vi "Fetch VI Method Info.vi"(8 "Error in":errorcluster caption="Error in (no error)", 9 "Dispatch (None)":T4, 10 "VI Reference":refnum<vi>, 11 "VI ProjectItem in":refnum<vi>) -> (0 "Error out":errorcluster, 3 "Method Spec Cluster":T1)   [LabVIEW 2023, in "VIDoc Parsing.lvlib"]
uses:
  VIDoc Parsing.lvlib
  TypeDefs/Class Dispatch Type Enum.ctl
  TypeDefs/Method Spec Cluster.ctl
  TypeDefs/VI Type Extended Enum.ctl
  <vilib>/picture/picture.llb/imagedata.ctl
  TypeDefs/Controls Info Cluster.ctl
  <vilib>/Utility/miscctls.llb/LVKeyTypeDef.ctl
  <vilib>/Utility/miscctls.llb/LVPointTypeDef.ctl
  Structure Reporter/Tree Cluster.ctl
  Structure Reporter/Structure Reporter.lvlib
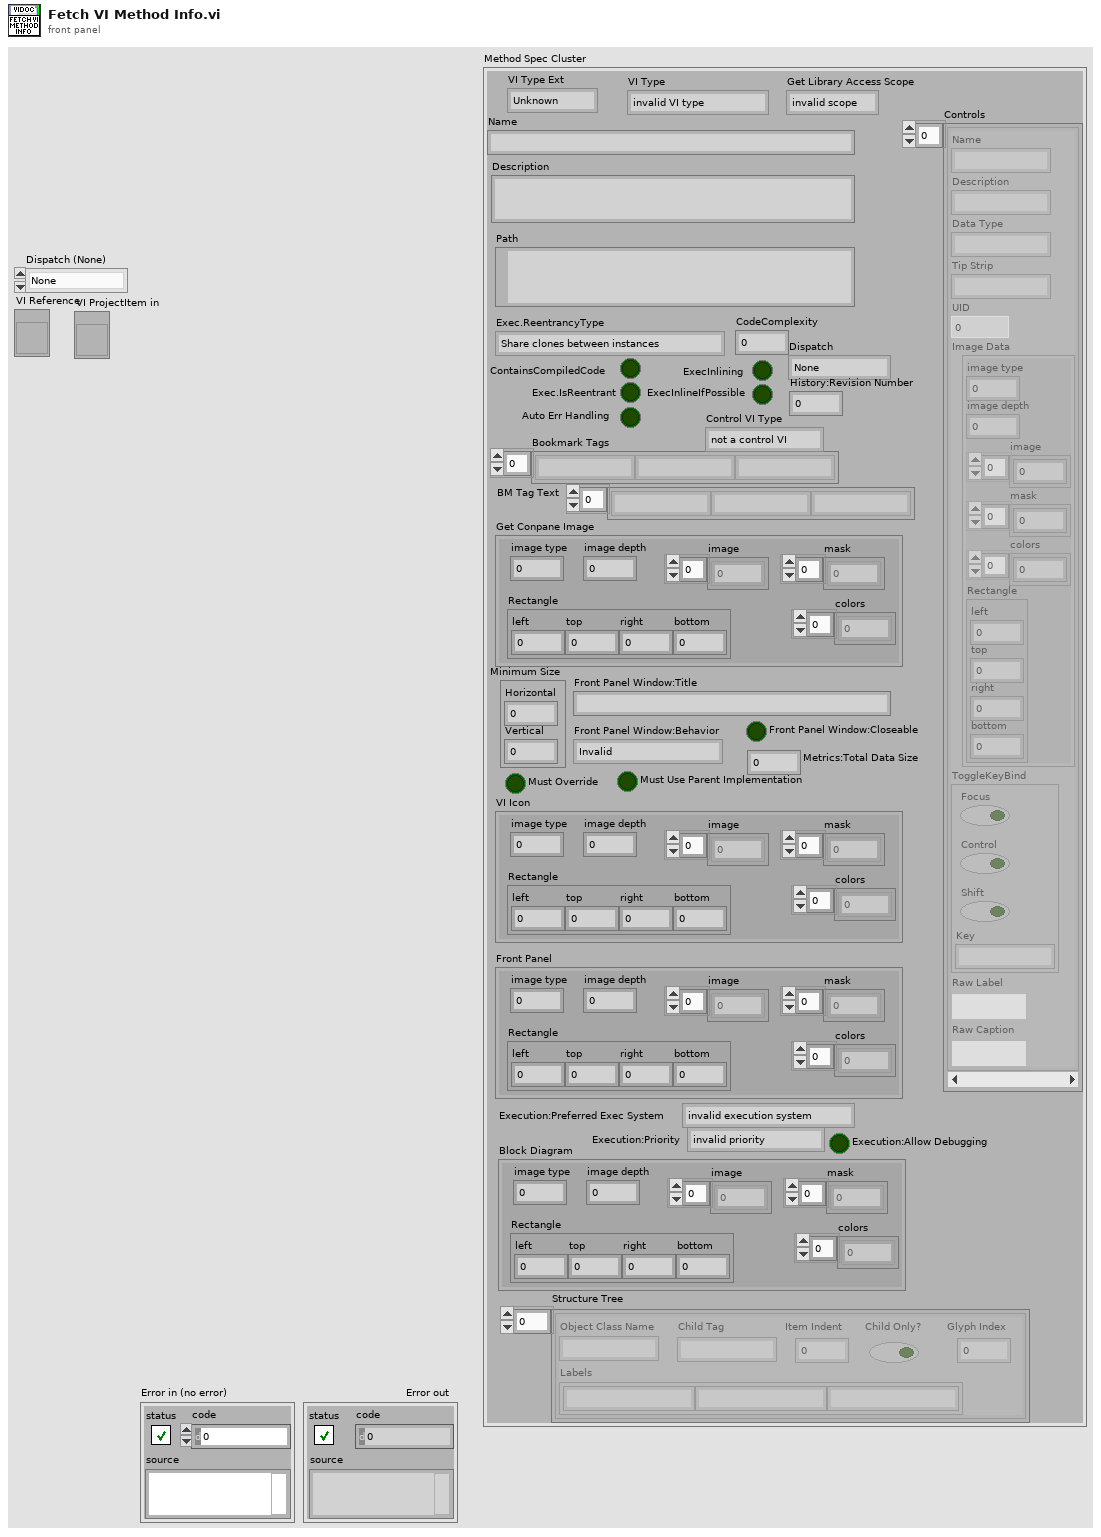
[diagram p1: front panel]
types:
  T1 = typedef "VIDoc Parsing.lvlib/Method Spec Cluster.ctl" = cluster{"VI Type Ext":T2, "Name":string, "Path":path, "Get Conpane Image":T3, "Description":string, "Get Library Access Scope":enum32{"invalid scope", "public", "private", "protected", "community"}, "Dispatch":T4, "ContainsCompiledCode":bool, "Exec.IsReentrant":bool, "Exec.ReentrancyType":enum16{"Share clones between instances", "Preallocate clone for each instance"}, "ExecInlining":bool, "ExecInlineIfPossible":bool, "Auto Err Handling":bool, "CodeComplexity":sgl, "Bookmark Tags":string[], "Control VI Type":enum32{"not a control VI", "control", "typedef", "strict typedef"}, "Controls":T5[], "VI Type":enum32{"invalid VI type", "Standard VI", "Control VI", "Global VI", "Polymorphic VI", "Configuration VI", "SubSystem", "Facade VI", "Method VI", "Statechart Diagram VI"}, "Minimum Size":T7, "Front Panel Window:Title":string, "Front Panel Window:Behavior":enum32{"Invalid", "Default", "Floating", "Floating/Auto-Hide", "Modal"}, "Front Panel Window:Closeable":bool, "Must Override":bool, "Must Use Parent Implementation":bool, "VI Icon":T3, "Front Panel":T3, "History:Revision Number":u32, "Metrics:Total Data Size":u32, "Execution:Allow Debugging":bool, "Execution:Preferred Exec System":enum32{"invalid execution system", "user interface", "standard", "instrument i/o", "data acquisition", "other 1", "other 2", "same as caller"}, "Execution:Priority":enum32{"invalid priority", "background priority", "normal priority", "above normal priority", "high priority", "time critical priority", "subroutine"}, "BM Tag Text":string[], "Block Diagram":T3, "Structure Tree":T8[]}
  T2 = typedef "VIDoc Parsing.lvlib/VI Type Extended Enum.ctl" = enum16{"Unknown", "Class Method", "Class Accessor Get", "Class Accessor Set", "Class Control", "Library Method", "Library Control", "VI", "Control"}
  T3 = typedef "imagedata.ctl" = cluster{"image type":i32, "image depth":i32, "image":u8[], "mask":u8[], "colors":u32[], "Rectangle":cluster{"left":i16, "top":i16, "right":i16, "bottom":i16}}
  T4 = typedef "VIDoc Parsing.lvlib/Class Dispatch Type Enum.ctl" = enum16{"None", "Static", "Dynamic"}
  T5 = typedef "VIDoc Parsing.lvlib/Controls Info Cluster.ctl" = cluster{"Name":string, "Description":string, "Data Type":string, "Tip Strip":string, "UID":i32, "Image Data":T3, "ToggleKeyBind":T6, "Raw Label":string, "Raw Caption":string}
  T6 = typedef "LVKeyTypeDef.ctl" = cluster{"Focus":bool, "Control":bool, "Shift":bool, "Key":string}
  T7 = typedef "LVPointTypeDef.ctl" = cluster{"Horizontal":i16, "Vertical":i16}
  T8 = typedef "VIDoc Parsing.lvlib/Structure Reporter.lvlib/Tree Cluster.ctl" = cluster{"Object Class Name":string, "Labels":string[], "Child Tag":string, "Item Indent":i32, "Child Only?":bool, "Glyph Index":i32}
  T9 = enum32{"not a control VI", "control", "typedef", "strict typedef"}
  T10 = enum16{"Share clones between instances", "Preallocate clone for each instance"}
  T11 = enum32{"invalid execution system", "user interface", "standard", "instrument i/o", "data acquisition", "other 1", "other 2", "same as caller"}
  T12 = enum32{"invalid priority", "background priority", "normal priority", "above normal priority", "high priority", "time critical priority", "subroutine"}
  T13 = enum32{"invalid scope", "public", "private", "protected", "community"}
  T14 = typedef "VIDoc Parsing.lvlib/Structure Reporter.lvlib/Structure Result 2.ctl" = cluster{"Depth":i32, "Top":i32, "Left":i32, "Frame index":i32, "Struct":i32, "Object Class Name":string, "Object UID":i32, "Label Visible":bool, "Object Label":string, "SD Label Visible":bool, "Object SD Label":string, "Frame Name":string, "Diag UID":i32, "Owner Class Name":string, "Owner UID":i32, "Diag Struct":i32[], "Parent Struct":i32, "Diag UIDs":i32[], "Tree Name":string, "Diag Ref":refnum<vi>, "Owner Classes":string[], "Owner":refnum<vi>, "Owner UIDs":i32[], "Tag Indent":i32, "Tag Value":i32, "Child Tag":string}
  T15 = typedef "LVBookmarkInfoTypeDef.ctl" = cluster{"Bookmark ID":u32, "Bookmark Tag":string, "Label Text":string}[]
  T16 = enum32{"Invalid", "Default", "Floating", "Floating/Auto-Hide", "Modal"}
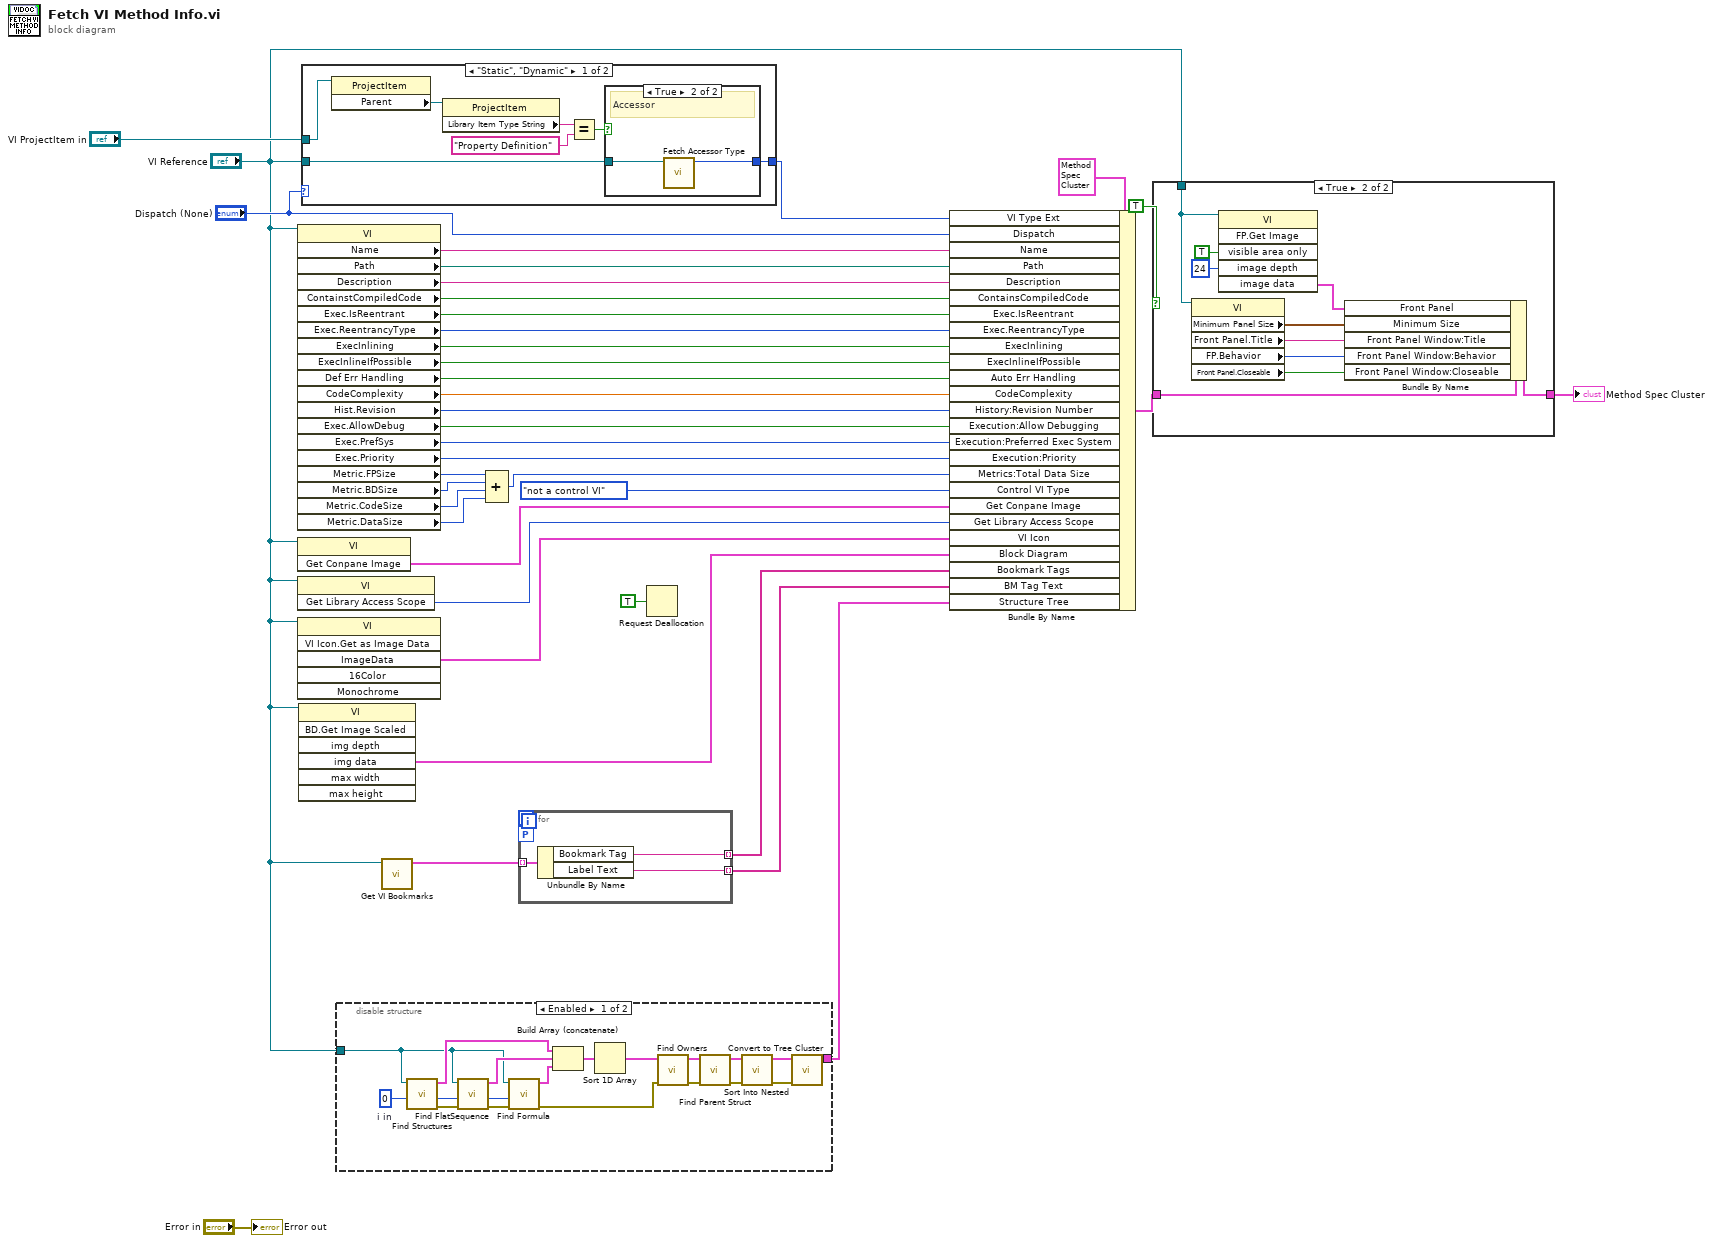
[diagram p0: block diagram]
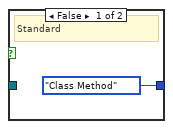
[diagram p4: hidden frame]
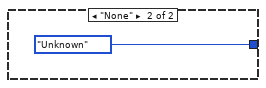
[diagram p5: hidden frame]
diagram:
  n1 = property class="VI"(reference="VI Reference") -> ("Name"=w31:string, "Path"=w30:path, "Description"=w29:string, "ContainstCompiledCode"=w28:bool, "Exec.IsReentrant"=w27:bool, "Exec.ReentrancyType"=w26:T10, "ExecInlining"=w25:bool, "ExecInlineIfPossible"=w24:bool, "Def Err Handling"=w23:bool, "CodeComplexity"=w22:sgl, "Hist.Revision"=w21:u32, "Exec.AllowDebug"=w20:bool, "Exec.PrefSys"=w19:T11, "Exec.Priority"=w18:T12, "Metric.FPSize"=w36:u32, "Metric.BDSize"=w35:u32, "Metric.CodeSize"=w34:u32, "Metric.DataSize"=w33:u32)  [unwired: 1 in, 2 out]
  n2 = invoke class="VI" method="Get Conpane Image"(reference="VI Reference") -> ("Get Conpane Image"=w16:T3)  [unwired: 2 in, 2 out]
  n3 = invoke class="VI" method="Get Library Access Scope"(reference="VI Reference") -> ("Get Library Access Scope"=w15:T13)  [unwired: 2 in, 2 out]
  n4 = invoke class="VI" method="VI Icon.Get as Image Data"(reference="VI Reference") -> ("ImageData"=w14:T3)  [unwired: 5 in, 5 out]
  n5 = invoke class="VI" method="BD.Get Image Scaled"(reference="VI Reference") -> ("img data"=w4:T3)  [unwired: 6 in, 6 out]
  n6 = case shown="\"Static\", \"Dynamic\"" "Dispatch (None)" {
    tunnel: "VI ProjectItem in" -> [w45 _]
    tunnel: [w41 VI_Type_Extended_Enum."Unknown" ("VI Type Ext")] -> w11
    tunnel: "VI Reference" -> [w39 _]
    frame "Static", "Dynamic" {
      n7 = property class="ProjectItem"(reference=w45) -> ("Parent"=w42:refnum<vi>)  [unwired: 1 in, 2 out]
      n8 = property class="ProjectItem"(reference=w42) -> ("Library Item Type String"=w43:string)  [unwired: 1 in, 2 out]
      n9 = Equal?(x=w43, y="Property Definition") -> (x = y?=w40:bool)
      n10 = case shown="True" w40 {
        tunnel: [VI_Type_Extended_Enum."Class Method" w47] -> w41
        tunnel: w39 -> [_ w48]
        frame False {
          # "Standard"
        }
        frame True {
          # "Accessor"
          n11 = call "Fetch Accessor Type.vi"("VI in"=w48) -> ("VI Type Ext"=w47:T2)  [unwired: 9 in, 1 out]
        }
      }
    }
    frame "None" {
    }
  }
  n12 = disable-structure "Diagram Disable Structure" shown="Enabled" {
    disable-tunnel: [w54 _] -> w3
    disable-tunnel: "VI Reference" -> [w50 _]
    frame Enabled {
      w67 = 0  # i in
      n13 = call "Find Structures.vi"("i in"=w67, "VI in"=w50) -> ("error out"=w53:errorcluster, "i out"=w66:i32, "Structures"=w68:T14[])  [unwired: 7 in]
      n14 = call "Find FlatSequence.vi"("error in (no error)"=w53, "i in"=w66, "VI in"=w50) -> ("error out"=w52:errorcluster, "i out"=w63:i32, "FlatSequences"=w65:T14[])  [unwired: 6 in]
      n15 = call "Find Formula.vi"("error in (no error)"=w52, "i in"=w63, "VI in"=w50) -> ("error out"=w51:errorcluster, "Array"=w64:T14[])  [unwired: 6 in, 1 out]
      n16 = Build Array (concatenate)(w68, w65, w64) -> (w62:T14[])
      n17 = Sort 1D Array(array=w62) -> (sorted array=w61:T14[])
      n18 = call "Find Owners.vi"("error in (no error)"=w51, "Array in"=w61) -> ("error out"=w59:errorcluster, "Array out"=w60:T14[])  [unwired: 8 in]
      n19 = call "Find Parent Struct.vi"("error in (no error)"=w59, "Objects in"=w60) -> ("error out"=w57:errorcluster, "Found Parent Struct"=w58:T14[])  [unwired: 8 in]
      n20 = call "Sort Into Nested.vi"("error in (no error)"=w57, "Found Parent Struct"=w58) -> ("error out"=w56:errorcluster, "Nested Structures"=w55:T14[])  [unwired: 8 in]
      n21 = call "Convert to Tree Cluster.vi"("error in (no error)"=w56, "Array in"=w55) -> ("Array out"=w54:T8[])  [unwired: 8 in, 1 out]
    }
    frame Disabled {
    }
  }
  n22 = call "Get VI Bookmarks.vi"("VI in"="VI Reference") -> ("BookmarkInfo"=w10:T15)  [unwired: 9 in, 1 out]
  n23 = Compound Arithmetic op=ADD(w36, w35, w34, w33) -> (w17:u32)
  n24 = for {
    tunnel: w10 -> [w71] mode=indexing
    tunnel: [w70] -> w9 mode=indexing
    workers-P: _ -> [_]
    tunnel: [w69] -> w8 mode=indexing
    n25 = Unbundle By Name(w71) -> ("Bookmark Tag"=w70:string, "Label Text"=w69:string)
  }
  n26 = Request Deallocation(TRUE ("flag")) -> ()
  n27 = Bundle By Name(cluster=T1 {"VI Type Ext"=enum."Unknown", "Name"="", "Path"=path "", "Get Conpane Image"={"image type"=0, "image depth"=0, "image"=[], "mask"=[], "colors"=[], "Rectangle"={"left"=0, "top"=0, "right"=0, "bottom"=0}}, "Description"="", "Get Library Access Scope"=enum."invalid scope", "Dispatch"=enum."None", "ContainsCompiledCode"=FALSE, "Exec.IsReentrant"=FALSE, "Exec.ReentrancyType"=enum."Share clones between instances", "ExecInlining"=FALSE, "ExecInlineIfPossible"=FALSE, "Auto Err Handling"=FALSE, "CodeComplexity"=0.0, "Bookmark Tags"=[], "Control VI Type"=enum."not a control VI", "Controls"=[], "VI Type"=enum."invalid VI type", "Minimum Size"={"Horizontal"=0, "Vertical"=0}, "Front Panel Window:Title"="", "Front Panel Window:Behavior"=enum."Invalid", "Front Panel Window:Closeable"=FALSE, "Must Override"=FALSE, "Must Use Parent Implementation"=FALSE, "VI Icon"={"image type"=0, "image depth"=0, "image"=[], "mask"=[], "colors"=[], "Rectangle"={"left"=0, "top"=0, "right"=0, "bottom"=0}}, "Front Panel"={"image type"=0, "image depth"=0, "image"=[], "mask"=[], "colors"=[], "Rectangle"={"left"=0, "top"=0, "right"=0, "bottom"=0}}, "History:Revision Number"=0, "Metrics:Total Data Size"=0, "Execution:Allow Debugging"=FALSE, "Execution:Preferred Exec System"=enum."invalid execution system", "Execution:Priority"=enum."invalid priority", "BM Tag Text"=[], "Block Diagram"={"image type"=0, "image depth"=0, "image"=[], "mask"=[], "colors"=[], "Rectangle"={"left"=0, "top"=0, "right"=0, "bottom"=0}}, "Structure Tree"=[]}, "VI Type Ext"=w11, "Dispatch"="Dispatch (None)", "Name"=w31, "Path"=w30, "Description"=w29, "ContainsCompiledCode"=w28, "Exec.IsReentrant"=w27, "Exec.ReentrancyType"=w26, "ExecInlining"=w25, "ExecInlineIfPossible"=w24, "Auto Err Handling"=w23, "CodeComplexity"=w22, "History:Revision Number"=w21, "Execution:Allow Debugging"=w20, "Execution:Preferred Exec System"=w19, "Execution:Priority"=w18, "Metrics:Total Data Size"=w17, "Control VI Type"=T9."not a control VI", "Get Conpane Image"=w16, "Get Library Access Scope"=w15, "VI Icon"=w14, "Block Diagram"=w4, "Bookmark Tags"=w9, "BM Tag Text"=w8, "Structure Tree"=w3) -> (w7:T1)
  n28 = case shown="True" TRUE {
    tunnel: [w72 w82] -> w38
    tunnel: w7 -> [w72 w81]
    tunnel: "VI Reference" -> [_ w80]
    frame False {
    }
    frame True {
      n29 = property class="VI"(reference=w80) -> ("Minimum Panel Size"=w79:T7, "Front Panel.Title"=w75:string, "FP.Behavior"=w74:T16, "Front Panel.Closeable"=w73:bool)  [unwired: 1 in, 2 out]
      n30 = invoke class="VI" method="FP.Get Image"(reference=w80, "visible area only"=TRUE ("Visible Area Only"), "image depth"=24 ("Image Depth")) -> ("image data"=w76:T3)  [unwired: 3 in, 5 out]
      n31 = Bundle By Name(cluster=w81, "Front Panel"=w76, "Minimum Size"=w79, "Front Panel Window:Title"=w75, "Front Panel Window:Behavior"=w74, "Front Panel Window:Closeable"=w73) -> (w82:T1)
    }
  }
  "Method Spec Cluster" <- w38
  "Error out" <- "Error in"
